vi "Global_WC_Drive_LockAngle.vi"() -> ()   [LabVIEW 2017]
panel:
  in  "Lock Angle":bool
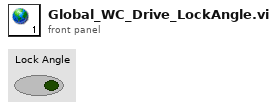
[diagram p1: front panel]
diagram:
